vi "Minify HTML.vi"(8 "error in (no error)":errorcluster, 11 "HTML in":string) -> (0 "error out":errorcluster, 3 "Minified HTML":string)   [LabVIEW 2019]
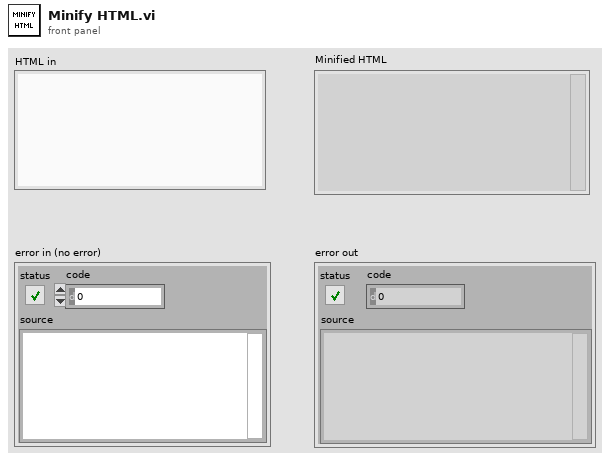
[diagram p1: front panel]
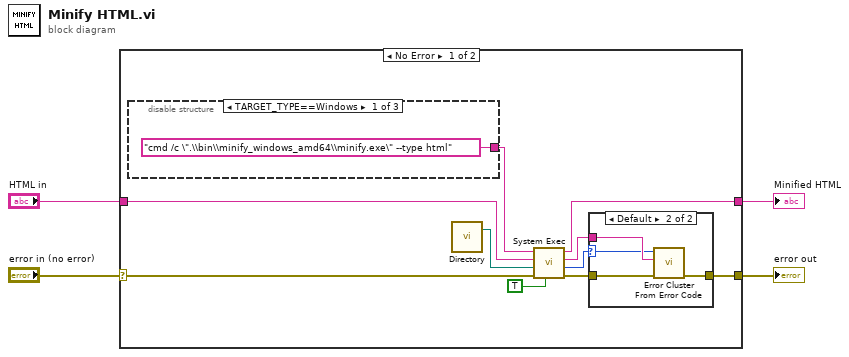
[diagram p0: block diagram]
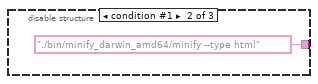
[diagram p2: hidden frame]
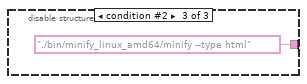
[diagram p3: hidden frame]
diagram:
  n1 = case shown="No Error" "error in (no error)" {
    selector: "error in (no error)" -> [w5 w24]
    tunnel: [w14 w23] -> w4
    tunnel: [w10 w24] -> w3
    tunnel: "HTML in" -> [w6 w23]
    frame No Error {
      n2 = disable-structure shown="TARGET_TYPE==Windows" {
        disable-tunnel: ["cmd /c \".\\bin\\minify_windows_amd64\\minify.exe\" --type html" ("command line (utility)") "./bin/minify_darwin_amd64/minify --type html" ("command line (utility)") "./bin/minify_linux_amd64/minify --type html" ("command line (utility)")] -> w7
        frame condition #0 (active) {
        }
        frame condition #1 {
        }
        frame condition #2 {
        }
      }
      n3 = call "Directory.vi"() -> ("Directory"=w12:path)  [unwired: 3 in]
      n4 = call <vilib>:"System Exec.vi"("run minimized? (F)"=TRUE, "error in (no error)"=w5, "working directory"=w12, "standard input"=w6, "command line"=w7) -> ("error out"=w11:errorcluster, "return code"=w8:i32, "standard error"=w9:string, "standard output"=w14:string)  [unwired: 1 in, 2 out]
      n5 = case shown="Default" w8 {
        selector: w8 -> [_ w19]
        tunnel: w11 -> [w18 w22]
        tunnel: [w18 w21] -> w10
        tunnel: w9 -> [_ w20]
        frame 0 {
        }
        frame Default {
          n6 = call <vilib>:"Error Cluster From Error Code.vi"("error in (no error)"=w22, "error message (\"\")"=w20, "error code (0)"=w19) -> ("error out"=w21:errorcluster)  [unwired: 6 in]
        }
      }
    }
    frame Error {
    }
  }
  "Minified HTML" <- w4
  "error out" <- w3
